vi "Full experiment AVI.vi"() -> ()   [LabVIEW 2018]
uses:
  <vilib>/userdefined/High Color/IMAQdx.ctl
  <vilib>/vision/Avi.llb/IMAQ AVI2 Codec Path.ctl
  <vilib>/Platform/TimedLoop/XDataNode/nitl_modes.ctl
  <vilib>/Platform/TimedLoop/XDataNode/timing_clust.ctl
  <vilib>/Platform/TimedLoop/XDataNode/wakeup.ctl
  <vilib>/platform/TimedLoop/XDataNode/XDataNode.xnode
  <vilib>/vision/driver/NI_Vision_Acquisition_Software.lvlib
  <vilib>/Platform/TimedLoop/XDataNode/XDNodeRunTimeDep.lvlib
panel:
  out "x-y":dbl
  out "Number of Frames":u32
  out "Array":string[](array[string])
  in  "Choose folder to save experiment videos":path
  in  "Rat ¹":i16
  out "Closing the experiment":bool
  out "Experiment":bool
  in  "Error massages":T1(tab)
  out "error message":string caption="Initialization error message"
  out "error message 2":string caption="Real time video-tracking error message"
  out "error message 3":string caption="Experiment video-tracking error message"
  out "error message 4":string caption="Closing the experiment error message"
  out "Real time video-tracking":bool
  out "Read LED Forward Bias in V":dbl
  out "Read LED Wavelength in nm":dbl
  out "Read Counts from machine":i32
  in  "Set Counts in amounts of counts\n(0 means INFINITY)":i32 format="%.0g"
  out "Read Duty Cycle from machine":i32
  in  "Set Duty Cycle in %":i32=5 format="%.0g"
  out "Read frequency from machine":i32
  in  "Set frequency in Hz":i32=20
  out "Read current from machine":dbl
  in  "Set current in ampere":sgl=1.0 caption="Set current in A"
  in  "Start experiment":bool
  in  "Stop experiment":bool
  out "Real Time image":T2(plugin-control)
  out "Initialization status":bool
  in  "Choose DC2100 Thorlabs":refnum<visa-resource-name>="ASRL0::INSTR" caption="resource name"
  in  "Choose camera":T3
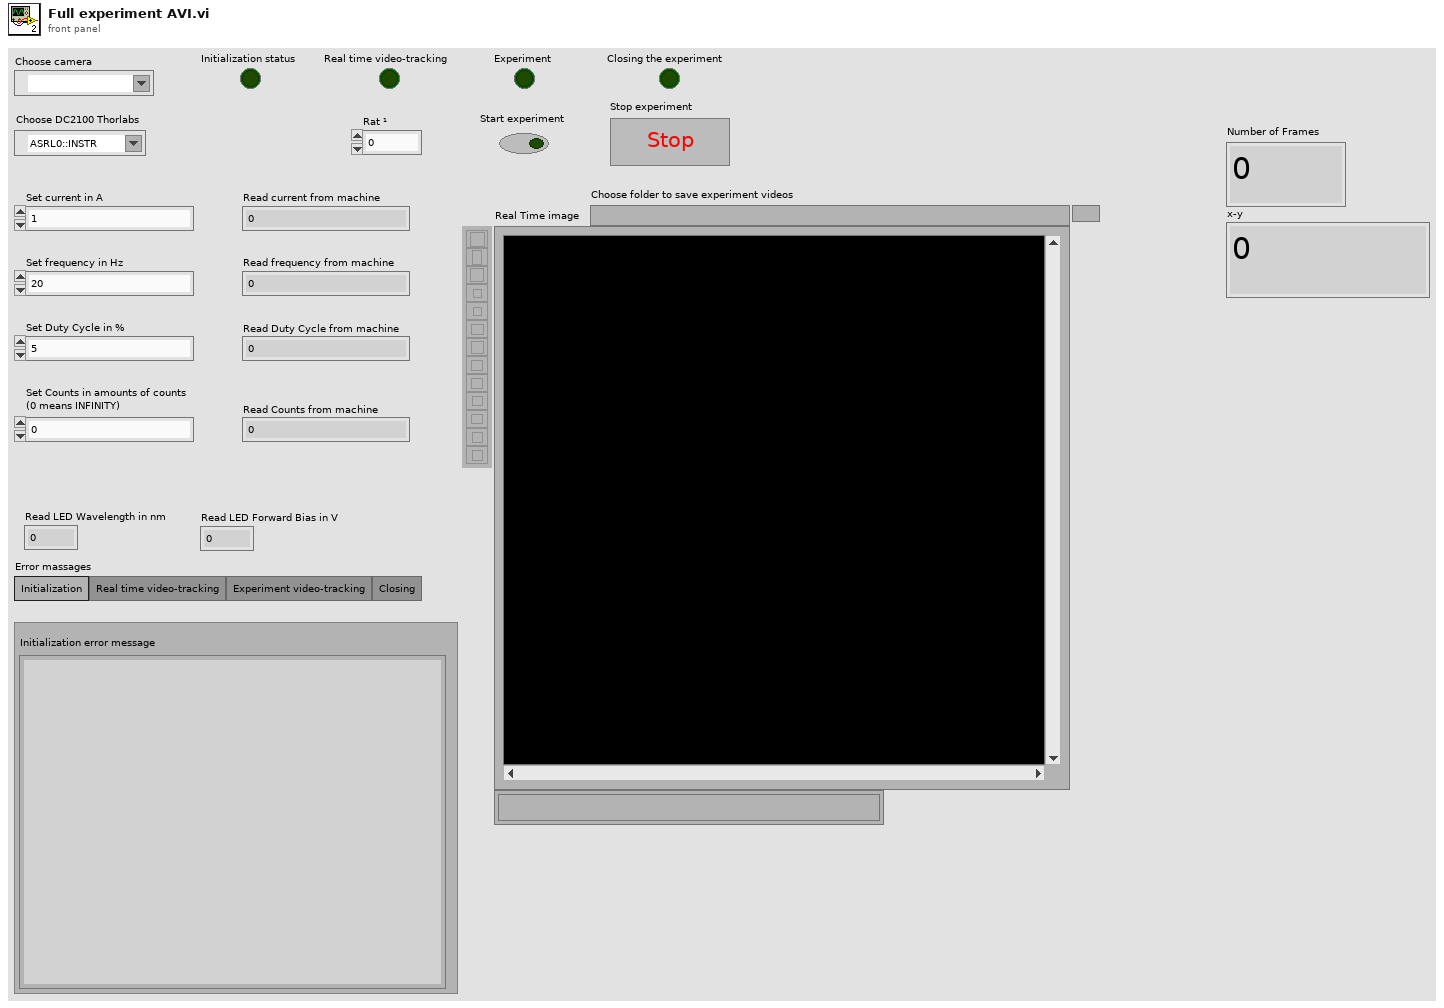
[diagram p1: front panel]
types:
  T1 = enum32{"Initialization", "Real time video-tracking", "Experiment video-tracking", "Closing"}
  T2 = typedef "IMAQ Image.ctl" = refnum<image>
  T3 = typedef "IMAQdx.ctl" = refnum<k21>
  T4 = typedef "XDNodeRunTimeDep.lvlib/nitl_modes.ctl" = enum32{"No Change", "Process missed periods, maintain original phase", "Discard missed periods, maintain original phase", "Process missed periods, ignore original phase", "Discard missed periods, ignore original phase"}
  T5 = typedef "XDNodeRunTimeDep.lvlib/timing_clust.ctl" = cluster{"Expected End [f-1]":u64, "Actual End [f-1]":u64, "Finished Late? [f-1]":bool, "Expected End [i-1]":u64, "Actual End [i-1]":u64, "Finished Late? [i-1]":bool, "Expected Start [i]":u64, "Actual Start [i]":u64, "Expected Start [f]":u64, "Actual Start [f]":u64, "Source Name":string, "Structure Name":string, "Period":i64, "Deadline":i64, "Offset":i64, "Start":i64, "Priority":i32, "Timeout":i32, "Mode":T4, "Wakeup Reason":T6, "Error":errorcluster, "Source Type":string, "Secondary Source Type":string, "Global End Time":u64, "Global Start Time":u64, "Frame Duration":u64, "Iteration Duration":u64, "Assigned CPU":i32, "I/O Scan Engine Mode":u32}
  T6 = typedef "XDNodeRunTimeDep.lvlib/wakeup.ctl" = enum32{"Normal", "Aborted", "Asynchronous wakeup", "Timing source error", "Timed loop error", "Timeout"}
  T7 = typedef "IMAQ AVI2 Codec Path.ctl" = u32
  T8 = typedef "IMAQ AVI2 Refnum.ctl" = refnum<k20>
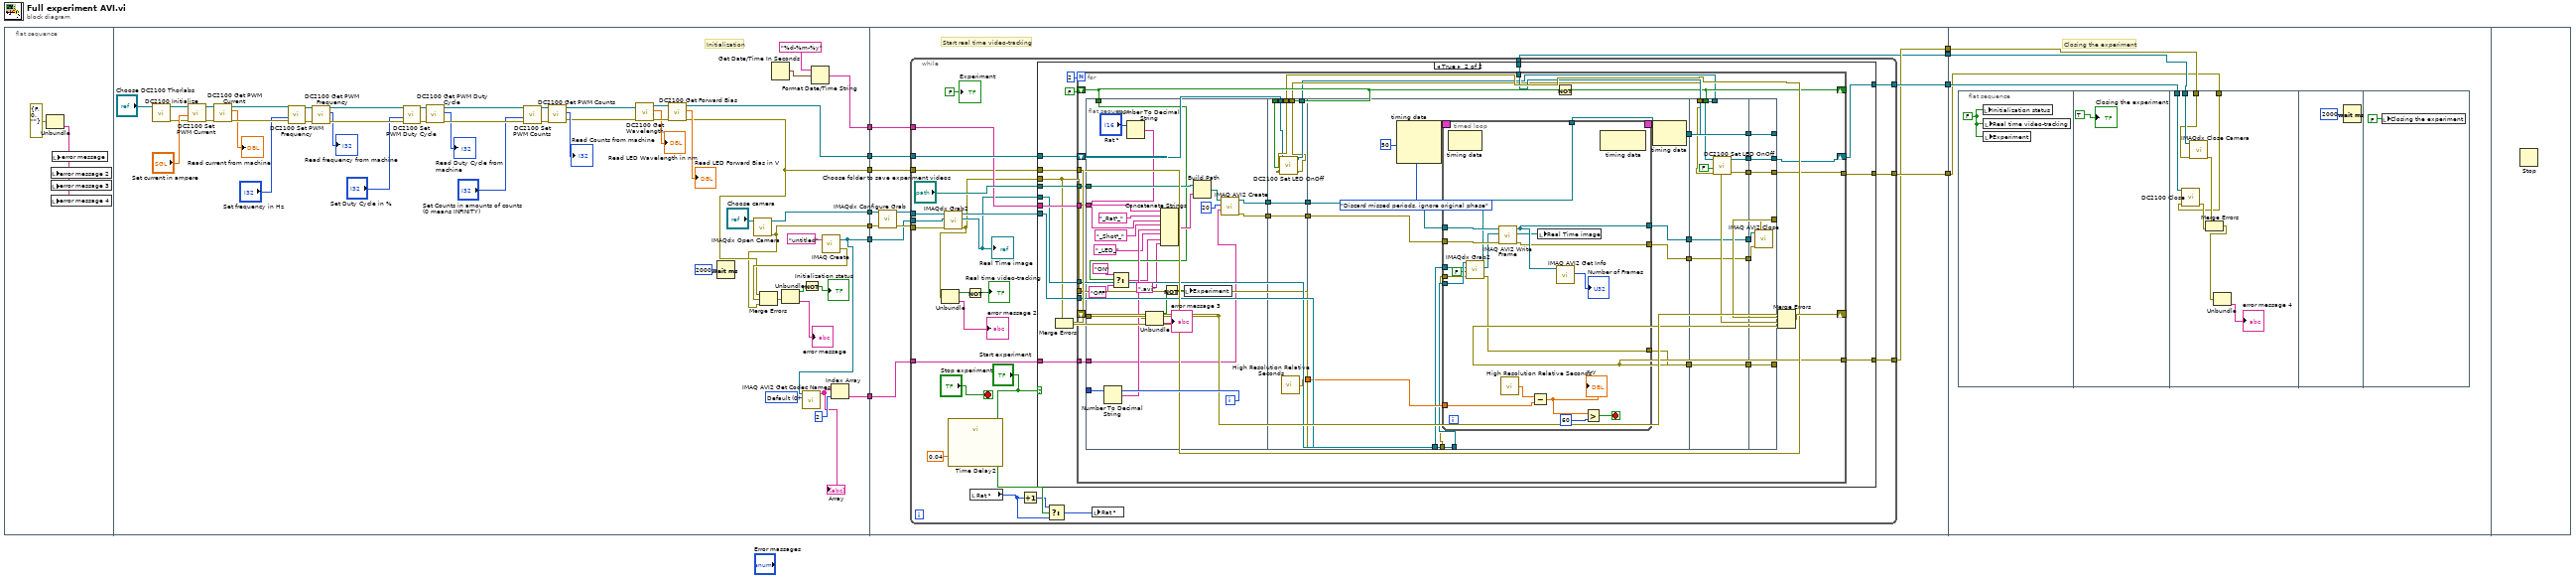
[diagram p0: block diagram]
diagram:
  n1 = flat-sequence {
    tunnel: [w61] -> w11
    tunnel: [w16] -> w10
    tunnel: [w28] -> w9
    tunnel: [w25] -> w8
    tunnel: [w20] -> w5
    tunnel: [w19] -> w4
    tunnel: [w15] -> w1
    tunnel: w11 -> [w77]
    tunnel: w10 -> [w74]
    tunnel: w9 -> [w73]
    tunnel: w8 -> [w72]
    tunnel: [w71] -> w7
    tunnel: [w66] -> w6
    tunnel: w5 -> [w70]
    tunnel: w4 -> [w69]
    tunnel: [w67] -> w3
    tunnel: [w68] -> w2
    tunnel: w1 -> [w65]
    tunnel: w7 -> [w247]
    tunnel: w6 -> [w246]
    tunnel: w3 -> [w245]
    tunnel: w2 -> [w244]
    frame #0 {
      n2 = Unbundle(errorcluster {"status"=FALSE, "code"=0, "source"=""} ("error constant")) -> ("source"=w12:string)  [unwired: 2 out]
      n3 = local write "error message 2"(w12) -> ()
      n4 = local write "error message 3"(w12) -> ()
      n5 = local write "error message 4"(w12) -> ()
      n6 = local write "error message"(w12) -> ()
    }
    frame #1 {
      w18 = T7 0 items=["Default", "System", "Built in Vision"] ("Codec Source")
      # "Initialization"
      n7 = call <instrlib>:"DC2100 Initialize.vi"("resource name"="Choose DC2100 Thorlabs") -> ("error out"=w32:errorcluster, "instrument handle out"=w33:refnum<visa-resource-name>)  [unwired: 9 in]
      n8 = call <instrlib>:"DC2100 Set PWM Current.vi"("error in (no error)"=w32, "Current (0.0)"="Set current in ampere", "instrument handle"=w33) -> ("error out"=w59:errorcluster, "instrument handle out"=w58:refnum<visa-resource-name>)  [unwired: 7 in]
      n9 = call <instrlib>:"DC2100 Get PWM Current.vi"("error in (no error)"=w59, "instrument handle"=w58) -> ("error out"=w49:errorcluster, "Current"=→"Read current from machine":dbl, "instrument handle out"=w50:refnum<visa-resource-name>)  [unwired: 7 in]
      n10 = call <instrlib>:"DC2100 Set PWM Frequency.vi"("error in (no error)"=w49, "Frequency (1)"="Set frequency in Hz", "instrument handle"=w50) -> ("error out"=w57:errorcluster, "instrument handle out"=w56:refnum<visa-resource-name>)  [unwired: 7 in]
      n11 = call <instrlib>:"DC2100 Get PWM Frequency.vi"("error in (no error)"=w57, "instrument handle"=w56) -> ("error out"=w47:errorcluster, "Frequency"=→"Read frequency from machine":i32, "instrument handle out"=w48:refnum<visa-resource-name>)  [unwired: 7 in]
      n12 = call <instrlib>:"DC2100 Set PWM Duty Cycle.vi"("error in (no error)"=w47, "Duty Cycle (1)"="Set Duty Cycle in %", "instrument handle"=w48) -> ("error out"=w55:errorcluster, "instrument handle out"=w54:refnum<visa-resource-name>)  [unwired: 7 in]
      n13 = call <instrlib>:"DC2100 Get PWM Duty Cycle.vi"("error in (no error)"=w55, "instrument handle"=w54) -> ("error out"=w45:errorcluster, "Duty Cycle"=→"Read Duty Cycle from machine":i32, "instrument handle out"=w46:refnum<visa-resource-name>)  [unwired: 7 in]
      n14 = call <instrlib>:"DC2100 Set PWM Counts.vi"("error in (no error)"=w45, "Counts (0)"="Set Counts in amounts of counts\n(0 means INFINITY)", "instrument handle"=w46) -> ("error out"=w53:errorcluster, "instrument handle out"=w52:refnum<visa-resource-name>)  [unwired: 7 in]
      n15 = call <instrlib>:"DC2100 Get PWM Counts.vi"("error in (no error)"=w53, "instrument handle"=w52) -> ("error out"=w29:errorcluster, "Counts"=→"Read Counts from machine":i32, "instrument handle out"=w30:refnum<visa-resource-name>)  [unwired: 7 in]
      n16 = call <instrlib>:"DC2100 Get Wavelength.vi"("error in (no error)"=w29, "instrument handle"=w30) -> ("error out"=w44:errorcluster, "Wavelength"=→"Read LED Wavelength in nm":dbl, "instrument handle out"=w43:refnum<visa-resource-name>)  [unwired: 7 in]
      n17 = call <instrlib>:"DC2100 Get Forward Bias.vi"("error in (no error)"=w44, "instrument handle"=w43) -> ("error out"=w20:errorcluster, "Forward Bias"=→"Read LED Forward Bias in V":dbl, "instrument handle out"=w28:refnum<visa-resource-name>)  [unwired: 7 in]
      n18 = Wait (ms)(milliseconds to wait=u32 2000) -> ()  [unwired: 1 out]
      n19 = call <vilib>:"IMAQdx Open Camera.vi"("Session In"="Choose camera") -> ("error out"=w19:errorcluster, "Session Out"=w61:T3)  [unwired: 9 in]
      n20 = Get Date/Time In Seconds() -> (seconds since 1Jan1904=w27:timestamp)
      n21 = Format Date/Time String(time format string (%c)="%d-%m-%y", seconds (now)=w27) -> (date/time string=w25:string)  [unwired: 1 in]
      n22 = call "IMAQ Create"("Image Name"="untitled") -> ("New Image"=w16:T2, "error out"=w21:errorcluster)  [unwired: 4 in]
      n23 = Merge Errors(w20, w21, w19) -> (w22:errorcluster)
      n24 = Unbundle(w22) -> ("status"=w23:bool, "source"=→"error message":string)  [unwired: 1 out]
      n25 = call "IMAQ AVI2 Get Codec Names"("Codec Source"=w18, "Image"=w16) -> ("Codec Names"=w14:string[])  [unwired: 8 in, 1 out]
      "Array" <- w14
      n26 = Not(x=w23) -> (.not. x?=→"Initialization status":bool)
      n27 = Index Array(array=w14, index=2) -> (element=w15:string)
    }
    frame #2 {
      # "Start real time video-tracking"
      n28 = call <vilib>:"IMAQdx Configure Grab.vi"("error in"=w69, "Session In"=w77) -> ("error out"=w76:errorcluster, "Session Out"=w75:T3)  [unwired: 8 in]
      n29 = while {
        tunnel: w76 -> [w102]
        tunnel: w75 -> [w101]
        tunnel: w74 -> [w100]
        tunnel: w73 -> [w96]
        tunnel: w72 -> [w94]
        tunnel: [w93] -> w71
        tunnel: w70 -> [w90]
        tunnel: [w89] -> w68
        tunnel: [w81] -> w67
        tunnel: [w80] -> w66
        tunnel: w65 -> [w79]
        stop <- "Stop experiment" stop-if-true
        n30 = call <vilib>:"IMAQdx Grab2.vi"("error in"=w102, "Image In"=w100, "Session In"=w101) -> ("error out"=w82:errorcluster, "Image Out"=w83:T2, "Session Out"=w84:T3)  [unwired: 5 in, 1 out]
        "Real Time image" <- w83
        n31 = Unbundle(w82) -> ("status"=w92:bool, "source"=→"error message 2":string)  [unwired: 1 out]
        n32 = call "Time Delay2"("Delay Time (s)"=0.04) -> ()  [unwired: 10 in, 1 out]
        n33 = Not(x=w92) -> (.not. x?=→"Real time video-tracking":bool)
        n34 = local read "Rat ¹"() -> (w85:i16)
        n35 = Increment(x=w85) -> (x+1=w87:i16)
        n36 = case shown="True" "Start experiment" {
          tunnel: w96 -> [w106 w117]
          tunnel: "Choose folder to save experiment videos" -> [_ w119]
          tunnel: w94 -> [_ w118]
          tunnel: [w106 w116] -> w93
          tunnel: w90 -> [w105 w111]
          tunnel: [w105 w115] -> w89
          tunnel: w84 -> [w103 w109]
          tunnel: w83 -> [_ w108]
          tunnel: w82 -> [w104 w107]
          tunnel: [w104 w114] -> w81
          tunnel: [w103 w113] -> w80
          tunnel: w79 -> [_ w112]
          frame False {
          }
          frame True {
            n37 = Merge Errors(w111, w107) -> (w110:errorcluster)
            n38 = for {
              N: 2 -> [_]
              shift-right: [w136] -> _
              shift-left: FALSE -> [w148]
              tunnel: w119 -> [w156]
              tunnel: w118 -> [w155]
              shift-right: [w153] -> _
              shift-left: w110 -> [w152]
              shift-right: [w133] -> w116
              shift-left: w117 -> [w143]
              tunnel: w111 -> [w144]
              tunnel: [w134] -> w115
              tunnel: [w139] -> w114
              tunnel: [w138] -> w113
              tunnel: w112 -> [w151]
              tunnel: w109 -> [w142]
              tunnel: w108 -> [w141]
              tunnel: w107 -> [w140]
              i -> [w154]
              n39 = flat-sequence {
                tunnel: w156 -> [w179]
                tunnel: w155 -> [w178]
                tunnel: w154 -> [w172]
                tunnel: w148 -> [w169]
                tunnel: w152 -> [w161]
                tunnel: w151 -> [w158]
                tunnel: [w164] -> w150
                tunnel: [w163] -> w149
                tunnel: w150 -> [w188]
                tunnel: w149 -> [w187]
                tunnel: w148 -> [w186]
                tunnel: [w188] -> w147
                tunnel: [w187] -> w146
                tunnel: [w181] -> w145
                tunnel: w144 -> [w185]
                tunnel: w143 -> [w184]
                tunnel: [w183] -> w135
                tunnel: [w182] -> w137
                tunnel: w147 -> [w202]
                tunnel: w146 -> [w201]
                tunnel: w145 -> [w200]
                tunnel: w142 -> [w199]
                tunnel: w141 -> [w198]
                tunnel: w140 -> [w197]
                tunnel: [w196] -> w131
                tunnel: [w195] -> w130
                tunnel: [w194] -> w129
                tunnel: [w193] -> w128
                tunnel: w131 -> [w229]
                tunnel: w130 -> [w230]
                tunnel: w129 -> [w236]
                tunnel: w128 -> [w235]
                tunnel: w137 -> [w234]
                tunnel: w136 -> [_]
                tunnel: w135 -> [w233]
                tunnel: [w236] -> w127
                tunnel: [w235] -> w126
                tunnel: [w232] -> w125
                tunnel: [w231] -> w124
                tunnel: [w230] -> w123
                tunnel: [w229] -> w122
                tunnel: [w237] -> w132
                tunnel: [w240] -> w133
                tunnel: [w241] -> w134
                tunnel: [w242] -> w138
                tunnel: [w243] -> w139
                tunnel: w127 -> [w243]
                tunnel: w126 -> [w242]
                tunnel: w125 -> [w241]
                tunnel: w124 -> [w240]
                tunnel: w123 -> [w239]
                tunnel: w122 -> [w238]
                frame #0 {
                  n40 = Number To Decimal String(number=w172) -> (decimal integer string=w171:string)  [unwired: 1 in]
                  n41 = Select(t="ON", s=w169, f="OFF") -> (s? t:f=w166:string)
                  n42 = Number To Decimal String(number="Rat ¹") -> (decimal integer string=w175:string)  [unwired: 1 in]
                  n43 = Unbundle(w161) -> ("status"=w160:bool, "source"=→"error message 3":string)  [unwired: 1 out]
                  n44 = Concatenate Strings(w178, "_Rat¹_" ("string"), w175, "_Shot¹_" ("string"), w171, "_LED_" ("string"), w166, ".avi" ("string")) -> (w174:string)
                  n45 = Not(x=w160) -> (.not. x?=w159:bool)
                  n46 = local write "Experiment"(w159) -> ()
                  n47 = Build Path(base path=w179, name or relative path=w174) -> (appended path=w180:path)
                  n48 = call "IMAQ AVI2 Create"("Codec"=w158, "Frames Per Second"=u32 20, "AVI Path"=w180) -> ("error out"=w163:errorcluster, "AVI Refnum"=w164:T8)  [unwired: 7 in]
                }
                frame #1 {
                  n49 = call <instrlib>:"DC2100 Set LED OnOff.vi"("error in (no error)"=w185, "LED On/Off (Off)"=w186, "instrument handle"=w184) -> ("error out"=w182:errorcluster, "instrument handle out"=w183:refnum<visa-resource-name>)  [unwired: 7 in]
                  n50 = call <vilib>:"High Resolution Relative Seconds.vi"() -> ("relative seconds"=w181:dbl)
                }
                frame #2 {
                  n51 = node-c288(i64 50 ("Period"), nitl_modes."Discard missed periods, ignore original phase" ("Mode")) -> (w192:T5)  [unwired: 1 in]
                  n52 = timed-loop {
                    tunnel: w202 -> [w218]
                    tunnel: w201 -> [w217]
                    tunnel: [w216] -> w196
                    tunnel: [w215] -> w195
                    tunnel: w200 -> [w213]
                    tunnel: w199 -> [w211]
                    tunnel: w198 -> [w210]
                    tunnel: w197 -> [w209]
                    tunnel: [w207] -> w194
                    tunnel: [w206] -> w193
                    timing: w192 -> [_]
                    timing-out: [_] -> w191
                    stop <- w219 stop-if-true
                    n53 = node-c288() -> ()  [unwired: 1 in, 1 out]
                    n54 = call <vilib>:"IMAQdx Grab2.vi"("error in"=w209, "Wait for Next Buffer? (Yes)"=FALSE, "Image In"=w210, "Session In"=w211) -> ("error out"=w207:errorcluster, "Image Out"=w208:T2, "Session Out"=w206:T3)  [unwired: 4 in, 1 out]
                    n55 = call "IMAQ AVI2 Write Frame"("error in (no error)"=w217, "Image"=w208, "AVI Refnum"=w218) -> ("error out"=w215:errorcluster, "Image Out (duplicate)"=w203:T2, "AVI Refnum (duplicate)"=w216:T8)  [unwired: 6 in]
                    n56 = call <vilib>:"High Resolution Relative Seconds.vi"() -> ("relative seconds"=w214:dbl)
                    n57 = Subtract(x=w214, y=w213) -> (x-y=w212:dbl)
                    "x-y" <- w212
                    n58 = local write "Real Time image"(w203) -> ()
                    n59 = call "IMAQ AVI2 Get Info"("AVI Refnum"=w216) -> ("Number of Frames"=→"Number of Frames":u32)  [unwired: 6 in, 4 out]
                    n60 = Greater?(x=w212, y=60) -> (0:w219:bool)
                    n61 = node-c288() -> ()  [unwired: 1 in, 1 out]
                  }
                  n62 = node-c288(w191) -> ()  [unwired: 1 out]
                }
                frame #3 {
                  n63 = call <instrlib>:"DC2100 Set LED OnOff.vi"("error in (no error)"=w234, "LED On/Off (Off)"=FALSE, "instrument handle"=w233) -> ("error out"=w232:errorcluster, "instrument handle out"=w231:refnum<visa-resource-name>)  [unwired: 7 in]
                }
                frame #4 {
                  n64 = call "IMAQ AVI2 Close"("error in (no error)"=w239, "AVI Refnum"=w238) -> ("error out"=w237:errorcluster)  [unwired: 9 in]
                }
              }
              n65 = Not(x=w148) -> (.not. x?=w136:bool)
              n66 = Merge Errors(w152, w132, w134, w139) -> (w153:errorcluster)
            }
          }
        }
        n67 = Select(t=w87, s="Start experiment", f=w85) -> (s? t:f=w86:i16)
        n68 = local write "Rat ¹"(w86) -> ()
        "Experiment" <- FALSE ("Experiment")
      }
    }
    frame #3 {
      # "Closing the experiment"
      n69 = flat-sequence {
        tunnel: w247 -> [w257]
        tunnel: w246 -> [w256]
        tunnel: w245 -> [w251]
        tunnel: w244 -> [w250]
        frame #0 {
          w248 = FALSE
          n70 = local write "Initialization status"(w248) -> ()
          n71 = local write "Real time video-tracking"(w248) -> ()
          n72 = local write "Experiment"(w248) -> ()
        }
        frame #1 {
          "Closing the experiment" <- TRUE
        }
        frame #2 {
          n73 = call <instrlib>:"DC2100 Close.vi"("error in (no error)"=w250, "instrument handle"=w257) -> ("error out"=w254:errorcluster)  [unwired: 9 in]
          n74 = call <vilib>:"IMAQdx Close Camera.vi"("error in"=w251, "Session In"=w256) -> ("error out"=w255:errorcluster)  [unwired: 9 in]
          n75 = Merge Errors(w255, w254) -> (w253:errorcluster)
          n76 = Unbundle(w253) -> ("source"=→"error message 4":string)  [unwired: 2 out]
        }
        frame #3 {
          n77 = Wait (ms)(milliseconds to wait=u32 2000) -> ()  [unwired: 1 out]
        }
        frame #4 {
          n78 = local write "Closing the experiment"(FALSE) -> ()
        }
      }
    }
    frame #4 {
      n79 = Stop() -> ()  [unwired: 1 in]
    }
  }
